vi "HFRR ADV v05.vi"() -> ()   [LabVIEW 2025] (continued)
          tunnel: w53 -> [w100]
          frame #0 {
            n17 = case shown="True" "Rd" {
              frame False {
              }
              frame True {
                n18 = while {
                  tunnel: "abcdefABCDEF" ("string 2") -> [w69]
                  shift-right: [w67] -> w61
                  shift-left: "" -> [w66]
                  i -> [w76]
                  stop <- w75 stop-if-true
                  n19 = Random Number (0-1)() -> (number: 0 to 1=w70:dbl)
                  n20 = Multiply(x=w70, y=62.0) -> (x*y=w72:dbl)
                  n21 = Decrement(x="Length 2") -> (x-1=w65:i16)
                  n22 = To Word Integer(number=w72) -> (16bit integer=w73:i16)
                  n23 = String Subset(string=w69, offset (0)=w73, length (rest)=1 ("length (rest)")) -> (substring=w68:string)
                  n24 = Greater Or Equal?(x=w76, y=w65) -> (x >= y?=w75:bool)
                  n25 = Concatenate Strings(w68, w66) -> (w67:string)
                }
                "String 10" <- w61
                n26 = local write "Rd"(FALSE ("Boolean 7")) -> ()
              }
            }
          }
          frame #1 {
            w88 = "_resized.jpg" ("command line")
            (unwired) ".jpg -resize 320x240 " ("string")
            (unwired) "Choose an Image File" ("prompt")
            # "-resize 1798x425"
            n27 = local read "Image Path"() -> (w82:path)
            n28 = Strip Path(path=w82) -> (stripped path=w77:path, name=w78:string)
            n29 = Match Pattern(string=w78, regular expression=".jpg") -> (before substring=→"before substring 2":string, after substring=→"after substring":string)  [unwired: 1 in, 2 out]
            n30 = Match Pattern(string=w78, regular expression="\\") -> (before substring=w84:string)  [unwired: 1 in, 3 out]
            n31 = Match Pattern(string=w84, regular expression=".jpg") -> (before substring=w83:string)  [unwired: 1 in, 3 out]
            n32 = Concatenate Strings("cmd /c convert " ("string"), w83, ".jpg -resize 320x240  " ("command line"), w83, w88) -> (w91:string)
            n33 = call <vilib>:"System Exec.vi"("run minimized? (F)"=TRUE, "wait until completion? (T)"=TRUE, "working directory"=w77, "command line"=w91) -> ("error out"=w90:errorcluster)  [unwired: 4 in, 3 out]
            "error out 2" <- w90
            n34 = Concatenate Strings(w83, w88) -> (w87:string)
          }
          frame #2 {
            n35 = Wait (ms)(milliseconds to wait=u32 2000 ("millisecond timer value")) -> (millisecond timer value=w96:u32)
          }
          frame #3 {
            n36 = case shown="No Error" w101 {
              tunnel: w102 -> [w105 _]
              tunnel: w100 -> [w103 _]
              frame No Error {
                (unwired) ".jpg" ("string")
                n37 = Path To String(path=w105) -> (string=w109:string)
                n38 = Concatenate Strings(w109, "\\" ("string"), w103) -> (w108:string)
                n39 = String To Path(string=w108) -> (path=w107:path)
                n40 = call <vilib>:"Read JPEG File.vi"("path to JPEG file"=w107) -> ("image data"=w111:T11)  [unwired: 8 in, 2 out]
                "image data" <- w111
                n41 = local write "Print 3"(FALSE ("Print 2")) -> ()
                n42 = call <vilib>:"Draw Flattened Pixmap.vi"("image data"=w111) -> ("new picture"=→"new picture":picture)  [unwired: 8 in]
              }
              frame Error {
              }
            }
          }
        }
      }
    }
    n43 = Wait (ms)(milliseconds to wait=u32 20 ("millisecond timer value")) -> ()  [unwired: 1 out]
    n44 = local read "Quit"() -> (w44:bool)
  }
  n45 = while {
    tunnel: w11 -> [_]
    stop <- w140 stop-if-true
    w131 = 1 ("y")
    # "New Adv Logics"
    n46 = local read "Main Tab"() -> (w138:T2)
    n47 = local read "Sign In"() -> (w127:bool)
    n48 = local read "Air Temperature"() -> (w117:bool)
    n49 = local read "Coefficient Of Friction"() -> (w118:bool)
    n50 = local read "USERNAME"() -> (w137:string)
    n51 = local read "Humidity"() -> (w116:bool)
    n52 = case shown="\"HOME\"" w138 {
      frame "HOME" {
        n53 = local write "main tab sub"(enum32{"Page 1", "Page 2"}."Page 1" ("main tab sub")) -> ()
      }
      frame Default {
        n54 = local write "main tab sub"(enum32{"Page 1", "Page 2"}."Page 2" ("main tab sub")) -> ()
      }
    }
    n55 = case shown="True" w127 {
      selector: w127 -> [_ w210]
      frame False {
      }
      frame True {
        n56 = Not(x=w210) -> (.not. x?=w209:bool)
        n57 = local write "Sign In"(w209) -> ()
        n58 = local write "Main Dashboard Buttons"(T1."Test Setup" ("Main Dashboard Buttons")) -> ()
      }
    }
    n59 = local read "USER ID"() -> (w134:string)
    n60 = case shown="\"Numeric Display\", Default" "Num/Graph" {
      frame "Numeric Display", Default {
        n61 = property on="Single/Multiple" class="RadioBtnsControl (strict)"("Visible"=FALSE) -> ()  [unwired: 2 in, 2 out]
        n62 = property on="Single - Graph" class="Ring (strict)"("Visible"=FALSE) -> ()  [unwired: 2 in, 2 out]
        n63 = local write "Main Tab Display"(T4."Dashboard 1" ("Main Tab Display")) -> ()
      }
      frame "Graph Display" {
        n64 = property on="Single/Multiple" class="RadioBtnsControl (strict)"("Visible"=TRUE) -> ()  [unwired: 2 in, 2 out]
        n65 = case shown="\"Multiple\"" "Single/Multiple" {
          frame "Single ", Default {
            n66 = property on="Single - Graph" class="Ring (strict)"("Visible"=TRUE) -> ()  [unwired: 2 in, 2 out]
            n67 = local write "Main Tab Display"(T4."Dashboard 3" ("Main Tab Display")) -> ()
          }
          frame "Multiple" {
            n68 = property on="Single - Graph" class="Ring (strict)"("Visible"=FALSE) -> ()  [unwired: 2 in, 2 out]
            n69 = local write "Main Tab Display"(T4."Dashboard 2" ("Main Tab Display")) -> ()
          }
        }
      }
    }
    n70 = local read "Stroke"() -> (w115:bool)
    n71 = call <vilib>:"Trim Whitespace.vi"("string"=w137) -> ("trimmed string"=w136:string)  [unwired: 1 in]
    n72 = call <vilib>:"Trim Whitespace.vi"("string"=w134) -> ("trimmed string"=w135:string)  [unwired: 1 in]
    n73 = case shown="True" w118 {
      selector: w118 -> [_ w161]
      frame False {
      }
      frame True {
        n74 = Not(x=w161) -> (.not. x?=w160:bool)
        n75 = local write "Coefficient Of Friction"(w160) -> ()
        n76 = local write "Tab Control 2"(T6."Coefficient Of Friction" ("Tab Control 2")) -> ()
      }
    }
    n77 = String Length(string=w136) -> (length=w133:i32)
    n78 = String Length(string=w135) -> (length=w132:i32)
    n79 = case shown="True" w117 {
      selector: w117 -> [_ w158]
      frame False {
      }
      frame True {
        n80 = Not(x=w158) -> (.not. x?=w156:bool)
        n81 = local write "Air Temperature"(w156) -> ()
        n82 = local write "Tab Control 2"(T6."Air Temperature" ("Tab Control 2")) -> ()
      }
    }
    n83 = case shown="True" w115 {
      selector: w115 -> [_ w152]
      frame False {
      }
      frame True {
        n84 = Not(x=w152) -> (.not. x?=w150:bool)
        n85 = local write "Stroke"(w150) -> ()
        n86 = local write "Tab Control 2"(T6."Stroke" ("Tab Control 2")) -> ()
      }
    }
    n87 = case shown="True" w116 {
      selector: w116 -> [_ w155]
      frame False {
      }
      frame True {
        n88 = Not(x=w155) -> (.not. x?=w153:bool)
        n89 = local write "Humidity"(w153) -> ()
        n90 = local write "Tab Control 2"(T6."Humidity" ("Tab Control 2")) -> ()
      }
    }
    n91 = case shown="\"Imaging\"" "Main Dashboard Buttons" {
      tunnel: [T2."HOME" ("Main Tab") T2."Test Setup" ("Main Tab") T2."Acquire" ("Main Tab") T2."Adv Scar" ("Main Tab") T2."Adv Scar Report" ("Main Tab") T2."Compare Files" ("Main Tab") T2."About" ("Main Tab")] -> w125
      frame "Home", Default {
      }
      frame "Test Setup" {
      }
      frame "Dashboard" {
      }
      frame "Imaging" {
      }
      frame "Report" {
      }
      frame "Analysis" {
      }
      frame "About" {
      }
    }
    n92 = Greater?(x=w133, y=w131) -> (0:w130:bool)
    n93 = Greater?(x=w132, y=w131) -> (0:w129:bool)
    n94 = And(x=w130, y=w129) -> (x .and. y?=w128:bool)
    n95 = case shown="False" w128 {
      frame False {
        n96 = property on="Sign In" class="Bool (strict)"("DisabledEnum"=T14."Disabled" ("Disabled")) -> ()  [unwired: 2 in, 2 out]
      }
      frame True {
        n97 = property on="Sign In" class="Bool (strict)"("DisabledEnum"=T14."Enabled" ("Disabled")) -> ()  [unwired: 2 in, 2 out]
      }
    }
    n98 = Wait (ms)(milliseconds to wait=u32 100) -> ()  [unwired: 1 out]
    n99 = local read "Main Tab Display"() -> (w119:T4)
    n100 = local write "Main Tab"(w125) -> ()
    n101 = case shown="\"Dashboard 3\"" w119 {
      frame "Dashboard 1", Default {
        n102 = property on="Reset Graph" class="Bool (strict)"("Visible"=FALSE) -> ()  [unwired: 2 in, 2 out]
      }
      frame "Dashboard 2" {
        n103 = property on="Reset Graph" class="Bool (strict)"("Visible"=TRUE) -> ()  [unwired: 2 in, 2 out]
      }
      frame "Dashboard 3" {
        n104 = property on="Reset Graph" class="Bool (strict)"("Visible"=TRUE) -> ()  [unwired: 2 in, 2 out]
      }
    }
    n105 = local read "Humidity"() -> (w122:bool)
    n106 = local read "Sample Temperature"() -> (w114:bool)
    n107 = local read "Air Temp vs Rh"() -> (w112:bool)
    n108 = local read "Frequency"() -> (w113:bool)
    n109 = case shown="True" w122 {
      frame False {
        n110 = local write "Humidity On Command"(TRUE ("Humidity On Command")) -> ()
        n111 = case shown="True" "Humidity Off Command" {
          selector: "Humidity Off Command" -> [_ w174]
          frame False {
          }
          frame True {
            n112 = Not(x=w174) -> (.not. x?=w173:bool)
            n113 = local write "Humidity Off Command"(w173) -> ()
            n114 = local read "WriteHumidity"() -> (w171:string[])
            n115 = local read "EVENT LOG"() -> (w168:string)
            n116 = call "Event Log.vi"("Content"="Humidity Control Off" ("string"), "EVENT LOG"=w168) -> ("EVENT LOG"=w169:string)  [unwired: 8 in, 1 out]
            n117 = Insert Into Array(array=w171, new element="R;1" ("new element/subarray")) -> (w172:string[])  [unwired: 1 in]
            n118 = local write "EVENT LOG"(w169) -> ()
            n119 = local write "WriteHumidity"(w172) -> ()
          }
        }
      }
      frame True {
        n120 = case shown="True" "Humidity On Command" {
          selector: "Humidity On Command" -> [_ w187]
          frame False {
          }
          frame True {
            n121 = local read "Set Rh"() -> (w182:dbl)
            n122 = Not(x=w187) -> (.not. x?=w186:bool)
            n123 = local write "Humidity On Command"(w186) -> ()
            n124 = Number To Fractional String(number=w182, precision (6)=i16 2) -> (F-format string=w179:string)  [unwired: 2 in]
            n125 = local read "WriteHumidity"() -> (w184:string[])
            n126 = Concatenate Strings("M;" ("new element/subarray"), w179) -> (w183:string)
            n127 = Concatenate Strings("Humidity Set to : " ("string"), w179, "% RH" ("string")) -> (w177:string)
            n128 = Insert Into Array(array=w184, new element=w183) -> (w185:string[])  [unwired: 1 in]
            n129 = disable-structure shown="Disabled" {
              disable-tunnel: w177 -> [w189 _]
              frame Disabled {
                n130 = local read "EVENT LOG"() -> (w190:string)
                n131 = call "Event Log.vi"("Content"=w189, "EVENT LOG"=w190) -> ("EVENT LOG"=w191:string)  [unwired: 8 in, 1 out]
                n132 = local write "EVENT LOG"(w191) -> ()
              }
              frame Enabled {
              }
            }
            n133 = local write "WriteHumidity"(w185) -> ()
          }
        }
        n134 = local write "Humidity Off Command"(TRUE ("Humidity Off Command")) -> ()
      }
    }
    n135 = local read "USERNAME"() -> (w121:string)
    n136 = local read "USER ID"() -> (w120:string)
    n137 = case shown="True" w113 {
      selector: w113 -> [_ w146]
      frame False {
      }
      frame True {
        n138 = Not(x=w146) -> (.not. x?=w144:bool)
        n139 = local write "Frequency"(w144) -> ()
        n140 = local write "Tab Control 2"(T6."Frequency" ("Tab Control 2")) -> ()
      }
    }
    n141 = case shown="True" w112 {
      selector: w112 -> [_ w143]
      frame False {
      }
      frame True {
        n142 = Not(x=w143) -> (.not. x?=w141:bool)
        n143 = local write "Air Temp vs Rh"(w141) -> ()
        n144 = local write "Tab Control 2"(T6."Air Temp vs Rh" ("Tab Control 2")) -> ()
      }
    }
    n145 = case shown="True" w114 {
      selector: w114 -> [_ w149]
      frame False {
      }
      frame True {
        n146 = Not(x=w149) -> (.not. x?=w147:bool)
        n147 = local write "Sample Temperature"(w147) -> ()
        n148 = local write "Tab Control 2"(T6."Sample Temperature" ("Tab Control 2")) -> ()
      }
    }
    n149 = local write "Operator ID"(w120) -> ()
    n150 = local write "tested by"(w121) -> ()
    n151 = local read "Quit"() -> (w140:bool)
    "Single" <- "Single - Graph"
  }
  n152 = flat-sequence {
    tunnel: ["ao0"] -> w14
    tunnel: w14 -> [w273]
    tunnel: [w271] -> w13
    tunnel: [w273] -> w12
    tunnel: [w275] -> w17
    tunnel: [w276] -> w43
    tunnel: w13 -> [w276]
    tunnel: w12 -> [w275]
    frame #0 {
    }
    frame #1 {
      w221 = FALSE ("Upld AR 2")
      # "kkkkk"
      # "C:\\Windows\\wndcm_pw_stdED hfrr.txt"
      # "C:\\LAB-IQ NXT"
      # "C:\\LAB-IQ NXT\\wndcm_pw_stdED hfrr.txt"
      # "password file"
      n153 = Current VI's Path() -> (path=w234:path)
      n154 = Strip Path(path=w234) -> (stripped path=w227:path)  [unwired: 1 out]
      n155 = Path To String(path=w227) -> (string=w229:string)
      n156 = local write "conststatus"(0.0 ("rpm value : 2")) -> ()
      n157 = local write "Upld AR 2"(TRUE ("Upld AR 2")) -> ()
      n158 = local write "Lan flag"(0.0 ("Lan flag")) -> ()
      n159 = local write "COUNT"(0 ("COUNT")) -> ()
      n160 = local write "FLAG 2"(0.0 ("FLAG 2")) -> ()
      n161 = local write "Com flag"(u32 0 ("Com flag")) -> ()
      n162 = local write "Re-Initialise"(TRUE ("Re-Initialise")) -> ()
      n163 = local write "refresh flag"(FALSE ("refresh flag")) -> ()
      n164 = local write "Json St Flg"(w221) -> ()
      n165 = Search/Split String(string=w229, search string/char (-)=".exe") -> (match + rest of string=w231:string)  [unwired: 1 in, 2 out]
      n166 = Match True/False String(2:".vi" ("false string"), 3:".exe" ("true string"), 4:w231) -> (0:w228:bool)  [unwired: 1 out]
      n167 = local write "Json End Flg"(w221) -> ()
      n168 = case shown="True" w228 {
        tunnel: w227 -> [w250 w252]
        tunnel: [w250 w251] -> w225
        frame False {
        }
        frame True {
          n169 = Strip Path(path=w252) -> (stripped path=w251:path)  [unwired: 1 out]
        }
      }
      n170 = Path To String(path=w225) -> (string=→"Gain path":string)
      n171 = local write "Main Tab Display"(T4."Dashboard 1" ("Main Tab Display")) -> ()
      n172 = local write "main tab sub"(enum32{"Page 1", "Page 2"}."Page 1" ("main tab sub")) -> ()
      n173 = local write "Main Tab"(T2."HOME" ("Main Tab")) -> ()
      n174 = local write "EVENT LOG"("") -> ()
      n175 = List Folder(path=path "C:/LAB-IQ-NXT" ("directory path"), pattern="*.txt") -> (filenames=w240:string[])  [unwired: 2 in, 3 out]
      n176 = Search 1D Array(1D array=w240, element="wndcm_pw_stdED hfrr.txt") -> (index of element=w243:i32)  [unwired: 1 in]
      n177 = Equal?(x=w243, y=-1) -> (x = y?=w238:bool)
      n178 = case shown="True" w238 {
        frame False {
        }
        frame True {
          n179 = String To Byte Array(string="123\n") -> (unsigned byte array=w257:u8[])
          n180 = Array Size(array=w257) -> (size(s)=w256:i32)
          n181 = for {
            N: w256 -> [_]
            tunnel: w257 -> [w270]
            tunnel: [w267] -> w259 mode=indexing
            tunnel: w256 -> [w262]
            i -> [w260]
            n182 = Decrement(x=w262) -> (x-1=w263:i32)
            n183 = Equal?(x=w260, y=w263) -> (x = y?=w264:bool)
            n184 = Index Array(array=w270, index=w260) -> (element=w269:u8)
            n185 = Number To Decimal String(number=w269) -> (decimal integer string=w268:string)  [unwired: 1 in]
            n186 = Select(t="", s=w264, f="\r") -> (s? t:f=w261:string)
            n187 = Concatenate Strings(w268, w261) -> (w267:string)
          }
          n188 = local read "file path"() -> (w253:path)
          n189 = Concatenate Strings(w259) -> (w255:string)
          n190 = call <vilib>:"Write Characters To File.vi"("append to file? (new file:F)"=FALSE, "character string"=w255, "file path (dialog if empty)"=w253) -> ()  [unwired: 2 in, 1 out]
        }
      }
      n191 = local write "clk"(0.0 ("clk")) -> ()
      n192 = local write "Flag"(0.0 ("Flag")) -> ()
      "file path" <- path "C:/LAB-IQ-NXT/wndcm_pw_stdED hfrr.txt" ("file path")
      "FF buffer" <- dbl[] [] ("FF buffer")
    }
    frame #2 {
      n193 = Wait (ms)(milliseconds to wait=u32 1000) -> (millisecond timer value=w271:u32)
    }
    frame #3 {
      n194 = local read "Re-Initialise"() -> (w274:bool)
      n195 = case shown="True" w274 {
        frame False {
        }
        frame True {
          n196 = local write "Re-Initialise"(FALSE ("Re-Initialise")) -> ()
        }
      }
    }
  }
  n197 = disable-structure shown="Disabled" {
    disable-tunnel: [w279 _] -> w19
    disable-tunnel: _ -> [w278 _]
    frame Disabled {
      n198 = while {
        tunnel: w278 -> [_]
        tunnel: [w280] -> w279
        tunnel: [w281] -> _
        i -> [w281]
        stop <- w280 stop-if-true
        w297 = u16 10 items=["1.0"=10, "1.5"=15, "2.0"=20] ("stop bits (10: 1 bit)")
        n199 = Wait (ms)(milliseconds to wait=u32 10) -> ()  [unwired: 1 out]
        n200 = call-poly "VISA Configure Serial Port"("VISA resource name"=refnum<visa-resource-name> "ASRL1::INSTR" ("COM PORT"), "timeout (10sec)"=u32 10, "baud rate (9600)"=u32 57600, "data bits (8)"=u16 8, "stop bits (10: 1 bit)"=w297) -> ("VISA resource name out"=w283:refnum<visa-resource-name>, "error out"=w292:errorcluster)  [unwired: 9 in]
        n201 = VISA Read(VISA resource name=w283, byte count=u32 2 ("byte count (0)")) -> (read buffer=w291:string)  [unwired: 1 in, 3 out]
        n202 = String Subset(string=w291, offset (0)=0, length (rest)=2 ("length (rest)")) -> (substring=w290:string)
        n203 = Match Pattern(string=w290, regular expression="<>") -> (offset past match=w287:i32)  [unwired: 1 in, 3 out]
        n204 = Greater Or Equal?(x=w287, y=0) -> (x >= y?=w282:bool)
        n205 = case shown="True" w282 {
          tunnel: w283 -> [_ w301]
          tunnel: w292 -> [_ w300]
          frame False {
          }
          frame True {
            n206 = VISA Read(VISA resource name=w301, byte count=u32 32 ("byte count (0)"), error in (no error)=w300) -> (read buffer=w299:string)  [unwired: 3 out]
            n207 = String Subset(string=w299, offset (0)=0, length (rest)=8 ("length (rest)")) -> (substring=w303:string)
            n208 = String Subset(string=w299, offset (0)=8, length (rest)=8 ("length (rest)")) -> (substring=w304:string)
            n209 = Decimal String To Number(string=w304) -> (number=w311:i32)  [unwired: 2 in, 1 out]
            n210 = Decimal String To Number(string=w303) -> (number=w307:i32)  [unwired: 2 in, 1 out]
            n211 = Divide(x=w311, y=10000) -> ()  [unwired: 1 out]
            n212 = Divide(x=w307, y=1000000) -> ()  [unwired: 1 out]
          }
        }
        n213 = local read "Quit"() -> (w280:bool)
      }
    }
    frame Enabled {
    }
  }
  n214 = local write "Err Count"(0 ("Err Count")) -> ()
  n215 = local write "FRICVALZ"(0.0 ("FRICVALZ")) -> ()
  n216 = Tick Count (ms)() -> (millisecond timer value=w32:u32)
  n217 = while {
    shift-right: [w330] -> w36
    shift-left: _ -> [w319]
    shift-right: [w329] -> w35
    shift-left: errorcluster {"status"=TRUE, "code"=0, "source"="Init"} ("error IO") -> [w321]
    shift-right: [w327] -> _
    shift-left: w32 -> [w328]
    tunnel: [w313] -> w23
    tunnel: [w326] -> _
    i -> [w326]
    stop <- w313 stop-if-true
    n218 = local read "Com Port 1"() -> (w320:refnum<visa-resource-name>)
    n219 = local read "Port 1a"() -> (w322:bool)
    n220 = local read "Port 3"() -> (w323:bool)
    n221 = Not Equal?(x=w320, y=w319) -> (x != y?=w318:bool)
    n222 = Or(x=w323, y=w322) -> (x .or. y?=w325:bool)
    n223 = Unbundle(w321) -> ("status"=→"Port 3":bool)  [unwired: 2 out]
    n224 = flat-sequence {
      tunnel: [w333] -> w317
      tunnel: w321 -> [w333]
      frame #0 {
        n225 = Wait (ms)(milliseconds to wait=u32 200) -> ()  [unwired: 1 out]
      }
    }
    n226 = case shown="False" w325 {
      frame False {
        w335 = FALSE ("Visible")
        n227 = property on="Port 1a" class="Bool (strict)"("Visible"=w335) -> ()  [unwired: 2 in, 2 out]
        n228 = property on="Port 3" class="Bool (strict)"("Visible"=w335) -> ()  [unwired: 2 in, 2 out]
      }
      frame True {
        w336 = TRUE ("Visible")
        n229 = property on="Port 1a" class="Bool (strict)"("Visible"=w336) -> ()  [unwired: 2 in, 2 out]
        n230 = property on="Port 3" class="Bool (strict)"("Visible"=w336) -> ()  [unwired: 2 in, 2 out]
      }
    }
    n231 = local read "Re-Initialise"() -> (w314:bool)
    n232 = Or(x=w318, y=w314) -> (x .or. y?=w315:bool)
    n233 = case shown="True" w315 {
      tunnel: [w331 errorcluster {"status"=TRUE, "code"=0, "source"="Init"} ("error out")] -> w316
      tunnel: w317 -> [w331 _]
      frame False {
      }
      frame True {
      }
    }
    n234 = case shown="No Error" w316 {
      selector: w316 -> [w337 w663]
      tunnel: [w342 w668] -> w330
      tunnel: [w341 w660] -> w329
      tunnel: w319 -> [w340 w666]
      tunnel: w328 -> [w339 w665]
      tunnel: [w338 w665] -> w327
      frame No Error {
        n235 = stacked-sequence {
          tunnel: [w352 _ _ _ _ _] -> w342
          tunnel: [w351 _ _ _ _ _] -> w341
          tunnel: w340 -> [w347 _ _ _ _ _]
          tunnel: w337 -> [w346 _ _ _ _ _]
          tunnel: w339 -> [_ w460 _ _ _ _]
          tunnel: [_ w459 _ _ _ _] -> w338
          tunnel: [_ w431 _ _ _ _] -> _
          frame #0 {
            n236 = property class="Instr"(reference=w347, error in=w346) -> (reference out=w349:refnum<visa-resource-name>, error out=w350:errorcluster, "Serial Settings:Number of Bytes at Serial Port"=w343:u32)
            "Sps 3" <- w343
            "Port 1" <- w343
            n237 = Greater?(x=w343, y=u32 5) -> (0:w345:bool)
            n238 = case shown="True" w345 {
              tunnel: w349 -> [w354 w375]
              tunnel: w350 -> [w353 w376]
              tunnel: [w353 w378] -> w351
              tunnel: [w354 w377] -> w352
              frame False {
              }
              frame True {
                # "Out as Volts"
                n239 = local read "Residual Uno"() -> (w369:string)
                n240 = while {
                  tunnel: [w415] -> w378
                  tunnel: [w414] -> w377
                  tunnel: w376 -> [w413]
                  tunnel: w375 -> [w412]
                  tunnel: [w409] -> _
                  shift-right: [w405] -> w357
                  shift-left: w369 -> [w407]
                  i -> [w409]
                  stop <- w410 stop-if-true
                  n241 = property class="Instr"(reference=w412, error in=w413) -> (reference out=w417:refnum<visa-resource-name>, error out=w416:errorcluster, "Serial Settings:Number of Bytes at Serial Port"=w408:u32)
                  n242 = VISA Read(VISA resource name=w417, byte count=w408, error in (no error)=w416) -> (VISA resource name out=w414:refnum<visa-resource-name>, read buffer=w406:string, error out=w415:errorcluster)  [unwired: 1 out]
                  n243 = Greater?(x=w408, y=u32 30) -> (0:w410:bool)
                  n244 = Concatenate Strings(w407, w406) -> (w405:string)
                }
                "UnoRead" <- w357
                n245 = while {
                  shift-right: [w391] -> w368
                  shift-left: w357 -> [w397]
                  tunnel: [w390] -> w364 mode=indexing
                  tunnel: [w392] -> _
                  i -> [w392]
                  stop <- w394 stop-if-true
                  n246 = Match Pattern(string=w397, regular expression="*") -> (after substring=w395:string)  [unwired: 1 in, 3 out]
                  n247 = Match Pattern(string=w395, regular expression="&") -> (before substring=w390:string, after substring=w391:string, offset past match=w393:i32)  [unwired: 1 in, 1 out]
                  n248 = Less Than 0?(x=w393) -> (x < 0?=w394:bool)
                }
                n249 = local write "Residual Uno"(w368) -> ()
                n250 = Array Size(array=w364) -> (size(s)=w365:i32)
                n251 = Decrement(x=w365) -> (x-1=w367:i32)
                n252 = Delete From Array(array=w364, length=1, index=w367) -> (array with subset deleted=w362:string[])  [unwired: 1 out]
                n253 = Array Size(array=w362) -> (size(s)=w361:i32)
                n254 = Decrement(x=w361) -> (x-1=w360:i32)
                n255 = while {
                  tunnel: [w389] -> w373 mode=indexing
                  tunnel: [w388] -> w372 mode=indexing
                  tunnel: w362 -> [w382] mode=indexing
                  tunnel: w360 -> [w381]
                  tunnel: [w379] -> _
                  i -> [w379]
                  stop <- w380 stop-if-true
                  w383 = 0 ("length (rest)")
                  w385 = ";" ("regular expression")
                  n256 = Less Or Equal?(x=w381, y=w379) -> (x <= y?=w380:bool)
                  n257 = Match Pattern(string=w382, regular expression=w385) -> (before substring=w387:string, after substring=w386:string)  [unwired: 1 in, 2 out]
                  n258 = Decimal String To Number(string=w387, default (0L)=w383) -> (number=w389:i32)  [unwired: 1 in, 1 out]
                  n259 = Match Pattern(string=w386, regular expression=w385) -> (before substring=w384:string)  [unwired: 1 in, 3 out]
                  n260 = Decimal String To Number(string=w384, default (0L)=w383) -> (number=w388:i32)  [unwired: 1 in, 1 out]
                }
                n261 = case shown="0, Default" "ADC Res" {
                  tunnel: [w400 w402] -> w356
                  frame 0, Default {
                    n262 = Divide(x=65535 ("length (rest)"), y=2 ("length (rest)")) -> (x/y=w400:dbl)
                  }
                  frame 1 {
                    n263 = Divide(x=16777216 ("length (rest)"), y=2 ("length (rest)")) -> (x/y=w402:dbl)
                  }
                }
                n264 = Bundle(w373, w372) -> (w363:cluster{i32[], i32[]})  [unwired: 1 in]
                n265 = Divide(x=w363, y=w356) -> (x/y=w374:cluster{dbl[], dbl[]})
                n266 = Multiply(x=w374, y=sgl 5.03 ("Numeric")) -> (x*y=w371:cluster{dbl[], dbl[]})
                n267 = Unbundle(w371) -> (→"Ch1":dbl[], →"Ch0":dbl[])
              }
            }
            n268 = Not(x=w345) -> (.not. x?=→"Port 1a":bool)
          }
          frame #1 {
            n269 = local read "zOff 2"() -> (w452:dbl)
            n270 = local read "Ch1"() -> (w442:dbl[])
            n271 = case shown="True" "Zero 2" {
              tunnel: w442 -> [_ w472]
              frame False {
              }
              frame True {
                n272 = call-poly <vilib>:"Mean.vi"("X"=w472) -> ("mean"=→"zOff 2":dbl)  [unwired: 1 out]
                n273 = local write "Zero 2"(FALSE ("Zero")) -> ()
              }
            }
            n274 = Subtract(x=w442, y=w452) -> (x-y=w448:dbl[])
            n275 = call-poly <vilib>:"Mean.vi"("X"=w442) -> ("mean"=w443:dbl)  [unwired: 1 out]
            "Slide 3" <- w443
            n276 = Multiply(x=w448, y=1.0 ("PG Oth")) -> (x*y=w434:dbl[])
            n277 = local read "FF buffer"() -> (w439:dbl[])
            n278 = Divide(x=w434, y=1) -> (x/y=w433:dbl[])
            "Fric Val" <- w433
            n279 = call <vilib>:"Mean PtByPt.vi"("x"=w443, "sample length"=10, "initialize"="Reset 2") -> ("mean"=→"Mean Pos Fil 2":dbl)  [unwired: 1 in, 1 out]
            n280 = Array Size(array=w439) -> (size(s)=w441:i32)
            n281 = call-poly <vilib>:"Mean.vi"("X"=w433) -> ("mean"=w447:dbl)  [unwired: 1 out]
            n282 = Insert Into Array(array=w439, index=w441, new element=w433) -> (w436:dbl[])
            n283 = Array Size(array=w436) -> (size(s)=w435:i32)
            n284 = case shown="True" "DC corr 2" {
              tunnel: w433 -> [w475 w478]
              tunnel: [w475 w477] -> w440
              tunnel: w447 -> [_ w476]
              frame False {
              }
              frame True {
                n285 = Subtract(x=w478, y=w476) -> (x-y=w477:dbl[])
              }
            }
            n286 = Tick Count (ms)() -> (millisecond timer value=w459:u32)
            n287 = Greater?(x=w435, y=1000) -> (0:w437:bool)
            n288 = Subtract(x=w459, y=w460) -> (x-y=w458:u32)
            n289 = case shown="True" w437 {
              tunnel: [w465 w468] -> w424
              tunnel: w436 -> [w465 w471]
              tunnel: w435 -> [_ w470]
              frame False {
              }
              frame True {
                n290 = Subtract(x=w470, y=1000) -> (x-y=w466:i32)
                n291 = Delete From Array(array=w471, length=w466, index=0) -> (array with subset deleted=w468:dbl[])  [unwired: 1 out]
              }
            }
            n292 = Divide(x=w458, y=u32 1000 ("x")) -> (x/y=w456:dbl)
            n293 = Array Size(array=w440) -> (size(s)=w455:i32)
            n294 = Divide(x=w455, y=w456) -> (x/y=w451:dbl)
            "Sps 2" <- w451
            n295 = Reciprocal(x=w451) -> (1/x=w449:dbl)
            "dt" <- w449
            n296 = local read "FRIC. FORCE :"() -> (w421:dbl)
            n297 = local write "FF buffer"(w424) -> ()
            n298 = Negate(x=w424) -> (-x=w423:dbl[])
            n299 = call "Elapsed Time5"("Time Target (s)"="check time s", "Reset"="Reset 3") -> ("Time has Elapsed"=w426:bool)  [unwired: 10 in, 7 out]
            n300 = Array Max & Min(array=w423) -> (max value=w431:dbl)  [unwired: 3 out]
            n301 = Bundle By Name("Y"=w440, "dt"=w449, "t0"=timestamp(0 s since 1904-01-01)) -> (w419:waveform(dbl))  [unwired: 1 in]
            n302 = Multiply(x=w421, y=21.1986) -> (x*y=w420:dbl)
            n303 = Greater Or Equal?(x=w431, y="Threshold value") -> (x >= y?=w427:bool)
            n304 = Multiply(x=w420, y=w419) -> (x*y=→"FF_Wfm":waveform(dbl))
            n305 = And(x=w427, y=w426) -> (x .and. y?=w425:bool)
            n306 = case shown="True" w425 {
              frame False {
                n307 = local write "Reset 3"(FALSE ("Reset 3")) -> ()
              }
              frame True {
                n308 = local write "Reset 3"(TRUE ("Reset 3")) -> ()
                n309 = local write "save dpt"(TRUE ("save dpt")) -> ()
              }
            }
          }
          frame #2 {
            n310 = local read "FF buffer"() -> (w485:dbl[])
            n311 = Array Max & Min(array=w485) -> (max value=w480:dbl, min value=w481:dbl)  [unwired: 2 out]
            n312 = Subtract(x=w480, y=w481) -> (x-y=w482:dbl)
            n313 = Multiply(x=1.0 ("y 2"), y="Threshold") -> ()  [unwired: 1 out]
            n314 = Greater?(x=w482, y="Threshold") -> (0:w479:bool)
            n315 = case shown="True" w479 {
              tunnel: w485 -> [_ w492]
              tunnel: [_ w490] -> _
              frame False {
              }
              frame True {
                w491 = 1.0 ("y")
                n316 = Delete From Array(array=w492, length=100, index=0) -> (deleted portion=w497:dbl[])  [unwired: 1 out]
                n317 = call-poly <vilib>:"Mean.vi"("X"=w497) -> ("mean"=w496:dbl)  [unwired: 1 out]
                n318 = Subtract(x=w492, y=w496) -> (x-y=w495:dbl[])
                n319 = Multiply(x=w491, y=w491) -> (x*y=w493:dbl)
                n320 = Multiply(x=w495, y=w493) -> (x*y=w494:dbl[])
                "FF cal val" <- w494
                n321 = Array Size(array=w494) -> (size(s)=w488:i32)
                n322 = Array Max & Min(array=w494) -> (max value=w487:dbl, min value=w486:dbl)  [unwired: 2 out]
                n323 = property on="FF Calibration g" class="WFGraph (strict)"("X Scale.Range:Minimum"=0.0 ("y"), "X Scale.Range:Maximum"=w488, "Y Scale.Range:Minimum"=w487, "Y Scale.Range:Maximum"=w486) -> ()  [unwired: 2 in, 2 out]
                n324 = local read "FRIC. FORCE :"() -> (w490:dbl)
              }
            }
          }
          frame #3 {
            # "5"
            n325 = local read "DISPLACEMENT :"() -> (w585:dbl)
            n326 = Multiply(x=w585, y=1.0) -> (x*y=w502:dbl)
            n327 = local read "zOff 3"() -> (w588:dbl)
            n328 = local read "Ch0"() -> (w515:dbl[])
            n329 = case shown="True" "Zero 3" {
              tunnel: w515 -> [_ w603]
              frame False {
              }
              frame True {
                n330 = call-poly <vilib>:"Mean.vi"("X"=w603) -> ("mean"=→"zOff 3":dbl)  [unwired: 1 out]
                n331 = local write "Zero 3"(FALSE ("Zero")) -> ()
              }
            }
            n332 = Add(x=w515, y="Offset") -> (x+y=w514:dbl[])
            n333 = Multiply(x=w502, y="DISPLACEMENT : 2") -> (x*y=w569:dbl)
            n334 = Subtract(x=w515, y=w588) -> (x-y=w572:dbl[])
            n335 = Multiply(x=w572, y=w569) -> (x*y=w571:dbl[])
            n336 = Multiply(x=w572, y=w502) -> (x*y=w584:dbl[])
            "ABS DP" <- w584
            n337 = local read "Standard Slip Gauge (mm)"() -> (w570:dbl)
            n338 = call-poly <vilib>:"Mean.vi"("X"=w571) -> ("mean"=w501:dbl)  [unwired: 1 out]
            "Disp (mm)" <- w501
            "software msrnt" <- w501
            n339 = Multiply(x=w514, y="Gain") -> (x*y=w509:dbl[])
            "Voltage LVDT Acq" <- w509
            "gLVDTraw" <- w509
            n340 = call-poly <vilib>:"Mean.vi"("X"=w584) -> ("mean"=w574:dbl)  [unwired: 1 out]
            n341 = case shown="True" "DC correction" {
              tunnel: w584 -> [w606 w609]
              tunnel: [w606 w608] -> w521
              tunnel: w574 -> [_ w607]
              frame False {
              }
              frame True {
                n342 = Subtract(x=w609, y=w607) -> (x-y=w608:dbl[])
              }
            }
            n343 = Divide(x=w501, y=w570) -> (x/y=w568:dbl)
            n344 = call-poly <vilib>:"Mean.vi"("X"=w509) -> ("mean"=w508:dbl)  [unwired: 1 out]
            n345 = Array Max & Min(array=w509) -> (max value=w513:dbl, min value=w512:dbl)  [unwired: 2 out]
            n346 = Multiply(x=w568, y=w569) -> (x*y=→"DISPLACEMENT : 3":dbl)
            n347 = Subtract(x=w513, y=w512) -> (x-y=→"Pk-Pk":dbl)
            n348 = local read "dt"() -> (w587:dbl)
            n349 = Threshold 1D Array(2:0.0 ("threshold y"), 3:w521) -> (0:w538:dbl)  [unwired: 1 in]
            n350 = Bundle By Name("Y"=w521, "dt"=w587, "t0"=timestamp(0 s since 1904-01-01)) -> (w576:waveform(dbl))  [unwired: 1 in]
            n351 = local read "FF_Wfm"() -> (w575:waveform(dbl))
            n352 = Equal To 0?(x=w538) -> (x = 0?=w539:bool)
            n353 = case shown="True" w539 {
              tunnel: w521 -> [_ w597]
              tunnel: [w593 w594] -> w534
              tunnel: w538 -> [w593 _]
              frame False {
              }
              frame True {
                n354 = Threshold 1D Array(1:20 ("start index (0)"), 2:0.0 ("threshold y"), 3:w597) -> (0:w594:dbl)
              }
            }
            n355 = call-poly <vilib>:"Extract Single Tone Information.vi"("time signal in"=w576) -> ("detected amplitude"=w510:dbl, "detected frequency"=→"Freq":dbl)  [unwired: 5 in, 4 out]
            n356 = Build Array(w576, w575) -> (w557:waveform(dbl)[])
            "Waveform Graph 2" <- w557
            n357 = Subtract(x=w508, y="LvdtOff") -> (x-y=w507:dbl)
            n358 = Subtract(x=w507, y=w510) -> (x-y=w519:dbl)
            n359 = Add(x=w510, y=w507) -> (x+y=w518:dbl)
            n360 = Index Array(array=w557) -> (element #1=w558:waveform(dbl), element #2=w560:waveform(dbl))  [unwired: 2 in]
            n361 = Multiply(x=w510, y=2.0) -> (x*y=w577:dbl)
            "Stroke" <- w577
            "Mean(RAW) Stroke" <- w577
            n362 = Bundle(w507, w519, w518) -> (→"Slide 8":cluster{dbl, dbl, dbl})  [unwired: 1 in]
            n363 = Unbundle By Name(w558) -> ("Y"=w531:dbl[])
            n364 = Split 1D Array(array=w521, index=w534) -> (second subarray=w535:dbl[])  [unwired: 1 out]
            n365 = In Range and Coerce(upper limit=1.5, x=w577, lower limit=0.5) -> (In Range?=w581:bool)  [unwired: 1 out]
            n366 = Split 1D Array(array=w531, index="Window") -> (second subarray=w549:dbl[])  [unwired: 1 out]
            n367 = Unbundle By Name(w560) -> ("Y"=w532:dbl[])
            n368 = Threshold 1D Array(1:180 ("start index (0)"), 2:0.0 ("threshold y"), 3:w535) -> (0:w533:dbl)
            n369 = local read "Test \nStatus"() -> (w578:bool)
            n370 = Split 1D Array(array=w532, index=w534) -> (second subarray=w529:dbl[])  [unwired: 1 out]
            n371 = Not(x=w581) -> (.not. x?=w580:bool)
            n372 = call-poly <vilib>:"RMS.vi"("X"=w549) -> ("rms value"=w505:dbl)  [unwired: 1 out]
            "Current (A)" <- w505
            n373 = Array Max & Min(array=w549) -> (max value=w563:dbl, min value=w564:dbl)  [unwired: 2 out]
            n374 = Array Max & Min(array=w532) -> (max value=w561:dbl, min value=w562:dbl)  [unwired: 2 out]
            n375 = Subtract(x=w563, y=w564) -> (x-y=w565:dbl)
            n376 = Subtract(x=w561, y=w562) -> (x-y=w566:dbl)
            n377 = And(x=w580, y=w578) -> (x .and. y?=w579:bool)
            n378 = Split 1D Array(array=w535, index=w533) -> (first subarray=w528:dbl[])  [unwired: 1 out]
            n379 = Split 1D Array(array=w529, index=w533) -> (first subarray=w526:dbl[])  [unwired: 1 out]
            n380 = case shown="True" w579 {
              tunnel: [i32[] [] w599] -> _
              frame False {
              }
              frame True {
                n381 = local read "UnoRead"() -> (w601:string)
                n382 = local read "Array"() -> (w602:string[])
                n383 = Build Array (concatenate)(w602, w601) -> (w600:string[])
                "Array" <- w600
                n384 = String Length(string=w600) -> (length=w599:i32[])
              }
            }
            n385 = local read "G_val"() -> (w551:dbl)
            n386 = Divide(x=w566, y=w565) -> (x/y=w554:dbl)
            n387 = call-poly <vilib>:"RMS.vi"("X"=w526) -> ("rms value"=w550:dbl)  [unwired: 1 out]
            n388 = call-poly <vilib>:"Hanning Window.vi"("X"=w528) -> ("Windowed X"=w527:dbl[])  [unwired: 1 out]
            n389 = call-poly <vilib>:"Hanning Window.vi"("X"=w526) -> ("Windowed X"=w525:dbl[])  [unwired: 1 out]
            n390 = local read "Constant (G)"() -> (w543:dbl)
            n391 = Divide(x=w550, y=w505) -> (x/y=w544:dbl)
            n392 = Build Array(w527, w525) -> (→"Waveform Graph 4":dbl[][])
            n393 = Multiply(x=w554, y=0.2) -> (x*y=w556:dbl)
            n394 = Multiply(x=0.8 ("y"), y=w551) -> (x*y=w555:dbl)
            n395 = Add(x=w556, y=w555) -> (x+y=w523:dbl)
            n396 = Multiply(x=w544, y=0.2) -> (x*y=w545:dbl)
            n397 = Multiply(x=0.8 ("y"), y=w543) -> (x*y=w546:dbl)
            n398 = Add(x=w545, y=w546) -> (x+y=w542:dbl)
            "Constant (G)" <- w542
            n399 = Not A Number/Path/Refnum?(number/path/refnum=w523) -> (NaN/Path/Refnum?=w522:bool)
            n400 = Select(t=0.0, s=w522, f=w523) -> (s? t:f=w503:dbl)
            "G_val" <- w503
            n401 = Multiply(x=w505, y=w503) -> (x*y=→"Friction Force (N)":dbl)
            n402 = Bundle(w542, "t"=w503) -> (→"pk-pk":cluster{dbl, "t":dbl})  [unwired: 1 in]
          }
          frame #4 {
            # "C:\\WinDucom\\data\\"
            # "?C:\\LAB-IQ-NXT\\data"
            n403 = case shown="True" "save dpt" {
              frame False {
              }
              frame True {
                n404 = local write "save dpt"(FALSE ("Hold 3")) -> ()
                n405 = local read "file count"() -> (w613:i32)
                n406 = Number To Decimal String(number=w613) -> (decimal integer string=w619:string)  [unwired: 1 in]
                n407 = Add(x=1, y=w613) -> (x+y=w614:i32)
                n408 = local write "file count"(w614) -> ()
                n409 = local read "FILE 2"() -> (w618:string)
                n410 = Concatenate Strings(w618, w619) -> (w611:string)
                n411 = Concatenate Strings("C:\\LAB-IQ-NXT\\data" ("Substring"), w611) -> (w626:string)
                n412 = local read "FF buffer"() -> (w621:dbl[])
                n413 = local read "ABS DP"() -> (w620:dbl[])
                n414 = Concatenate Strings(w626, ".dpf" ("Substring")) -> (w624:string)
                n415 = Build Array(w621, w620) -> (w616:dbl[][])
                n416 = Concatenate Strings("FF ( V ); DP( mincron ) " ("character string"), "\r") -> (w630:string)
                n417 = String To Path(string=w624) -> (path=w622:path)
                n418 = Transpose 2D Array(2D array=w616) -> (transposed array=w615:dbl[][])
                n419 = call <vilib>:"Write Characters To File.vi"("append to file? (new file:F)"=FALSE, "character string"=w630, "file path (dialog if empty)"=w622) -> ("new file path (Not A Path if cancelled)"=w627:path)  [unwired: 2 in]
                n420 = Array To Spreadsheet String(delimiter (Tab)=";", array=w615, 3:"" ("format string")) -> (spreadsheet string=w617:string)
                "String 9" <- w617
                n421 = call <vilib>:"Write Characters To File.vi"("append to file? (new file:F)"=TRUE, "character string"=w617, "file path (dialog if empty)"=w627) -> ()  [unwired: 2 in, 1 out]
              }
            }
          }
          frame #5 {
            n422 = case shown="True" "Hold 4" {
              frame False {
              }
              frame True {
                n423 = File Dialog(6:"*.dpf" ("pattern"), 11:path "C:/LAB-IQ-NXT" ("start path")) -> (0:w637:errorcluster, 3:w652:path)  [unwired: 5 in, 2 out]
                n424 = Unbundle(w637) -> ()  [unwired: 3 out]
                n425 = call <vilib>:"Read Characters From File.vi"("file path (dialog if empty)"=w652) -> ("character string"=w642:string)  [unwired: 5 in, 3 out]
                n426 = Spreadsheet String To Array(delimiter (Tab)=";", format string="%S", spreadsheet string=w642, array type (2D Dbl)=string[][] []) -> (array=w646:string[][])
                n427 = for {
                  tunnel: w646 -> [w656] mode=indexing
                  tunnel: [w655] -> w647 mode=indexing
                  n428 = for {
                    tunnel: w656 -> [w658] mode=indexing
                    tunnel: [w657] -> w655 mode=indexing
                    n429 = call <vilib>:"Trim Whitespace.vi"("string"=w658) -> ("trimmed string"=w657:string)  [unwired: 1 in]
                  }
                }
                n430 = Fract/Exp String To Number(string=w647) -> (number=w649:dbl[][])  [unwired: 3 in, 1 out]
                n431 = Array Subset(array=w649, index (row)=1 ("index (col)")) -> (w651:dbl[][])  [unwired: 3 in]
                n432 = Index Array(array=w651, index (col) #1=0 ("disabled index (col)"), index (col) #2=1 ("disabled index (col)")) -> (element #1=w640:dbl[], element #2=w639:dbl[])  [unwired: 2 in]
                n433 = Build Array(w640, w639) -> (→"Waveform Graph":dbl[][])
              }
            }
          }
        }
      }
      frame Error {
        w674 = u16 0 items=["None", "XON/XOFF", "RTS/CTS", "XON/XOFF & RTS/CTS", "DTR/DSR", "XON/XOFF & DTR/DSR"] ("flow control (0:none)  2")
        w672 = u16 10 items=["1.0"=10, "1.5"=15, "2.0"=20] ("stop bits 2")
        w670 = u16 0 items=["None", "Odd", "Even", "Mark", "Space"] ("parity 2")
        w671 = u32 10000  # timeout (10sec)
        n434 = VISA Close(VISA resource name=w666, error in (no error)=w663) -> (error out=w667:errorcluster)
        n435 = local write "Sps 3"(0.0 ("Sps 4")) -> ()
        n436 = call <vilib>:"Clear Errors.vi"("error in (no error)"=w667) -> ("error out"=w664:errorcluster)  [unwired: 5 in, 1 out]
        n437 = local read "Com Port 1"() -> (w659:refnum<visa-resource-name>)
        n438 = call-poly "VISA Configure Serial Port"("VISA resource name"=w659, "timeout (10sec)"=w671, "baud rate (9600)"=u32 250000 ("baud rate  2"), "data bits (8)"=u16 8 ("data bits  2"), "parity (0:none)"=w670, "error in (no error)"=w664, "stop bits (10: 1 bit)"=w672, "flow control (0:none)"=w674) -> ("VISA resource name out"=w675:refnum<visa-resource-name>, "error out"=w676:errorcluster)  [unwired: 6 in]
        n439 = flat-sequence {
          tunnel: w675 -> [w678]
          tunnel: w676 -> [w677]
          tunnel: [w678] -> w668
          tunnel: [w677] -> w660
          frame #0 {
            n440 = Wait (ms)(milliseconds to wait=u32 50) -> ()  [unwired: 1 out]
          }
        }
        "Residual Uno" <- ""
        "Port 1 Error" <- w660
      }
    }
    n441 = local read "Quit"() -> (w313:bool)
    "Error Uno" <- w321
  }
  n442 = while {
    shift-right: [w695] -> w16
    shift-left: _ -> [w686]
    shift-right: [w694] -> w15
    shift-left: errorcluster {"status"=FALSE, "code"=0, "source"="Init"} ("error out") -> [w688]
    tunnel: [w680] -> w22
    tunnel: [w693] -> _
    i -> [w693]
    stop <- w680 stop-if-true
    n443 = local read "Com Port 2"() -> (w687:refnum<visa-resource-name>)
    n444 = local read "Port 2a"() -> (w689:bool)
    n445 = local read "Port 4"() -> (w690:bool)
    n446 = Not Equal?(x=w687, y=w686) -> (x != y?=w685:bool)
    n447 = Or(x=w690, y=w689) -> (x .or. y?=w692:bool)
    n448 = Unbundle(w688) -> ("status"=→"Port 4":bool)  [unwired: 2 out]
    n449 = flat-sequence {
      tunnel: w688 -> [w699]
      tunnel: [w699] -> w684
      frame #0 {
        n450 = Wait (ms)(milliseconds to wait=u32 50) -> ()  [unwired: 1 out]
      }
    }
    n451 = local read "Re-Initialise"() -> (w681:bool)
    n452 = case shown="True" w692 {
      frame False {
        w700 = FALSE ("Visible")
        n453 = property on="Port 2a" class="Bool (strict)"("Visible"=w700) -> ()  [unwired: 2 in, 2 out]
        n454 = property on="Port 4" class="Bool (strict)"("Visible"=w700) -> ()  [unwired: 2 in, 2 out]
      }
      frame True {
        w701 = TRUE ("Visible")
        n455 = property on="Port 2a" class="Bool (strict)"("Visible"=w701) -> ()  [unwired: 2 in, 2 out]
        n456 = property on="Port 4" class="Bool (strict)"("Visible"=w701) -> ()  [unwired: 2 in, 2 out]
      }
    }
    n457 = Or(x=w685, y=w681) -> (x .or. y?=w682:bool)
    n458 = case shown="True" w682 {
      tunnel: [w696 errorcluster {"status"=TRUE, "code"=0, "source"="Init"} ("error out")] -> w683
      tunnel: w684 -> [w696 _]
      frame False {
      }
      frame True {
      }
    }
    n459 = case shown="Error" w683 {
      selector: w683 -> [w702 w856]
      tunnel: [w704 w861] -> w695
      tunnel: [w703 w854] -> w694
